vi "All Integration Tests.vi"(8 "error in (no error)":errorcluster) -> (0 "error out":errorcluster)   [LabVIEW 2026, in "Tests.lvlib"]
doc: "Aggregator for the Lumberjack unit tier. Holds every pure-VI unit test as a parallel subVI so the whole tier runs from one call. Has no assertions itself; each child registers its own via Define Test. Run directly for a fast, fixture-free unit-only pass (interactive Caraya dialog), or let Test.vi call it inside the suite for a headless, reported run. Add a unit test by dropping it here in parallel (Test-Strategy 3.2, 6)."
uses:
  Tests.lvlib
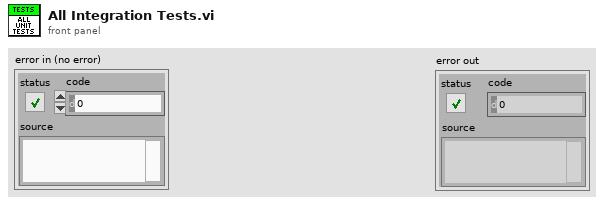
[diagram p1: front panel]
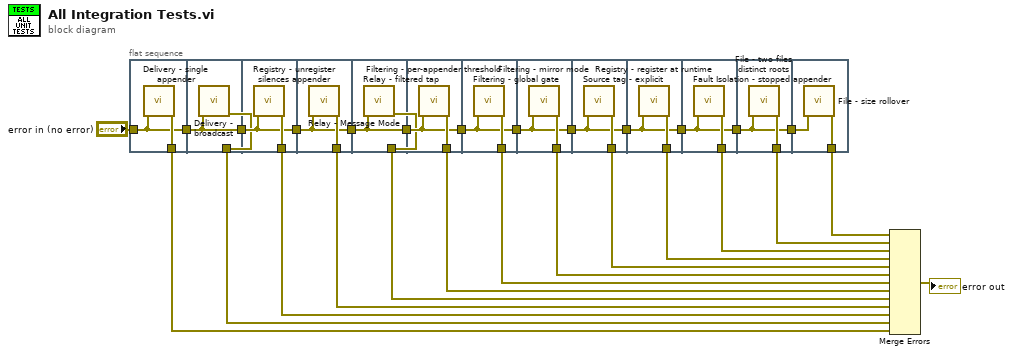
[diagram p0: block diagram]
diagram:
  n1 = flat-sequence {
    tunnel: "error in (no error)" -> [w28]
    tunnel: [w29] -> w3
    tunnel: [w28] -> w26
    tunnel: [w31] -> w27
    tunnel: w26 -> [w31]
    tunnel: [w30] -> _
    tunnel: [w30] -> w4
    tunnel: w27 -> [w32]
    tunnel: [w33] -> w5
    tunnel: [w32] -> w25
    tunnel: w25 -> [w34]
    tunnel: [w35] -> w6
    tunnel: [w34] -> w24
    tunnel: w24 -> [w37]
    tunnel: [w36] -> _
    tunnel: [w37] -> w21
    tunnel: [w36] -> w7
    tunnel: w21 -> [w38]
    tunnel: [w39] -> w8
    tunnel: [w38] -> w20
    tunnel: w20 -> [w40]
    tunnel: [w41] -> w9
    tunnel: [w40] -> w19
    tunnel: w19 -> [w42]
    tunnel: [w43] -> w10
    tunnel: [w42] -> w18
    tunnel: w18 -> [w44]
    tunnel: [w45] -> w11
    tunnel: [w44] -> w17
    tunnel: w17 -> [w46]
    tunnel: [w47] -> w12
    tunnel: [w46] -> w16
    tunnel: w16 -> [w48]
    tunnel: [w49] -> w13
    tunnel: [w48] -> w15
    tunnel: w15 -> [w50]
    tunnel: [w51] -> w14
    tunnel: [w50] -> w2
    tunnel: w2 -> [w53]
    tunnel: [w52] -> w1
    frame #0 {
      n2 = call "Delivery - single appender.vi"("error in (no error)"=w28) -> ("error out"=w29:errorcluster)  [unwired: 10 in]
    }
    frame #1 {
      n3 = call "Delivery - broadcast.vi"("error in (no error)"=w31) -> ("error out"=w30:errorcluster)  [unwired: 10 in]
    }
    frame #2 {
      n4 = call "Registry - unregister silences appender.vi"("error in (no error)"=w32) -> ("error out"=w33:errorcluster)  [unwired: 10 in]
    }
    frame #3 {
      n5 = call "Relay - Message Mode.vi"("error in (no error)"=w34) -> ("error out"=w35:errorcluster)  [unwired: 10 in]
    }
    frame #4 {
      n6 = call "Relay - filtered tap.vi"("error in (no error)"=w37) -> ("error out"=w36:errorcluster)  [unwired: 10 in]
    }
    frame #5 {
      n7 = call "Filtering - per-appender threshold.vi"("error in (no error)"=w38) -> ("error out"=w39:errorcluster)  [unwired: 10 in]
    }
    frame #6 {
      n8 = call "Filtering - global gate.vi"("error in (no error)"=w40) -> ("error out"=w41:errorcluster)  [unwired: 10 in]
    }
    frame #7 {
      n9 = call "Filtering - mirror mode.vi"("error in (no error)"=w42) -> ("error out"=w43:errorcluster)  [unwired: 10 in]
    }
    frame #8 {
      n10 = call "Source tag - explicit.vi"("error in (no error)"=w44) -> ("error out"=w45:errorcluster)  [unwired: 10 in]
    }
    frame #9 {
      n11 = call "Registry - register at runtime.vi"("error in (no error)"=w46) -> ("error out"=w47:errorcluster)  [unwired: 10 in]
    }
    frame #10 {
      n12 = call "Fault Isolation - stopped appender.vi"("error in (no error)"=w48) -> ("error out"=w49:errorcluster)  [unwired: 10 in]
    }
    frame #11 {
      n13 = call "File - two files distinct roots.vi"("error in (no error)"=w50) -> ("error out"=w51:errorcluster)  [unwired: 10 in]
    }
    frame #12 {
      n14 = call "File - size rollover.vi"("error in (no error)"=w53) -> ("error out"=w52:errorcluster)  [unwired: 10 in]
    }
  }
  n15 = Merge Errors(w1, w14, w13, w12, w11, w10, w9, w8, w7, w6, w5, w4, w3) -> (→"error out":errorcluster)
